vi "niFpga wdp fft butterfly.vi"(6 "enable":bool, 8 "index=0?":bool, 9 "twiddle factor":T1, 10 "data in 1":T2, 11 "data in 0":T2) -> (2 "data out 1":cluster{"y":fxp<+/-,11,2>, "y":fxp<+/-,11,2>}, 3 "data out 0":cluster{"y":fxp<+/-,11,2>, "y":fxp<+/-,11,2>})   [LabVIEW 2017]
uses:
  <vilib>/rvi/Analysis/measure/FFT/config/niFpgaFFTScalingScheme.ctl
  <vilib>/rvi/ClientSDK/Core/DevComputerLib/Private/FourWireProtocol(cint64).vi
  <vilib>/rvi/FXPMathLib/FxpAdd/XNode/nifxpmath_Add.xnode
  <vilib>/rvi/FXPMathLib/FxpSub/XNode/nifxpmath_Sub.xnode
  <vilib>/rvi/FXPMathLib/FxpMultComplex/XNode/niFpgaMultComplex.xnode
  <vilib>/rvi/FXPMathLib/SharedSubVIs/typedef/nifxpmath_BASIC_ImplementationSettings.ctl
  <vilib>/fxp/LVFixedPointQuantizationPolicyTypeDef.ctl
  <vilib>/fxp/LVFixedPointOverflowPolicyTypeDef.ctl
  <vilib>/rvi/FXPMathLib/FxpInterpret/XNode/nifxpmath_Interpret.xnode
  <vilib>/rvi/FXPMathLib/sim/FxpSim.dll
  <vilib>/rvi/ClientSDK/Core/DevComputerLib/niFpgaDevCompUtilities.lvlib
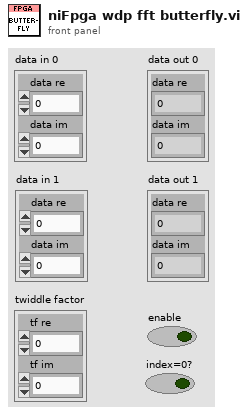
[diagram p1: front panel]
types:
  T1 = cluster{"tf re":fxp<+/-,16,2>, "tf im":fxp<+/-,16,2>}
  T2 = cluster{"data re":fxp<+/-,8,1>, "data im":fxp<+/-,8,1>}
  T3 = typedef "niFpgaFFTScalingScheme.ctl" = enum16{"Unscaled", "Scaled"}
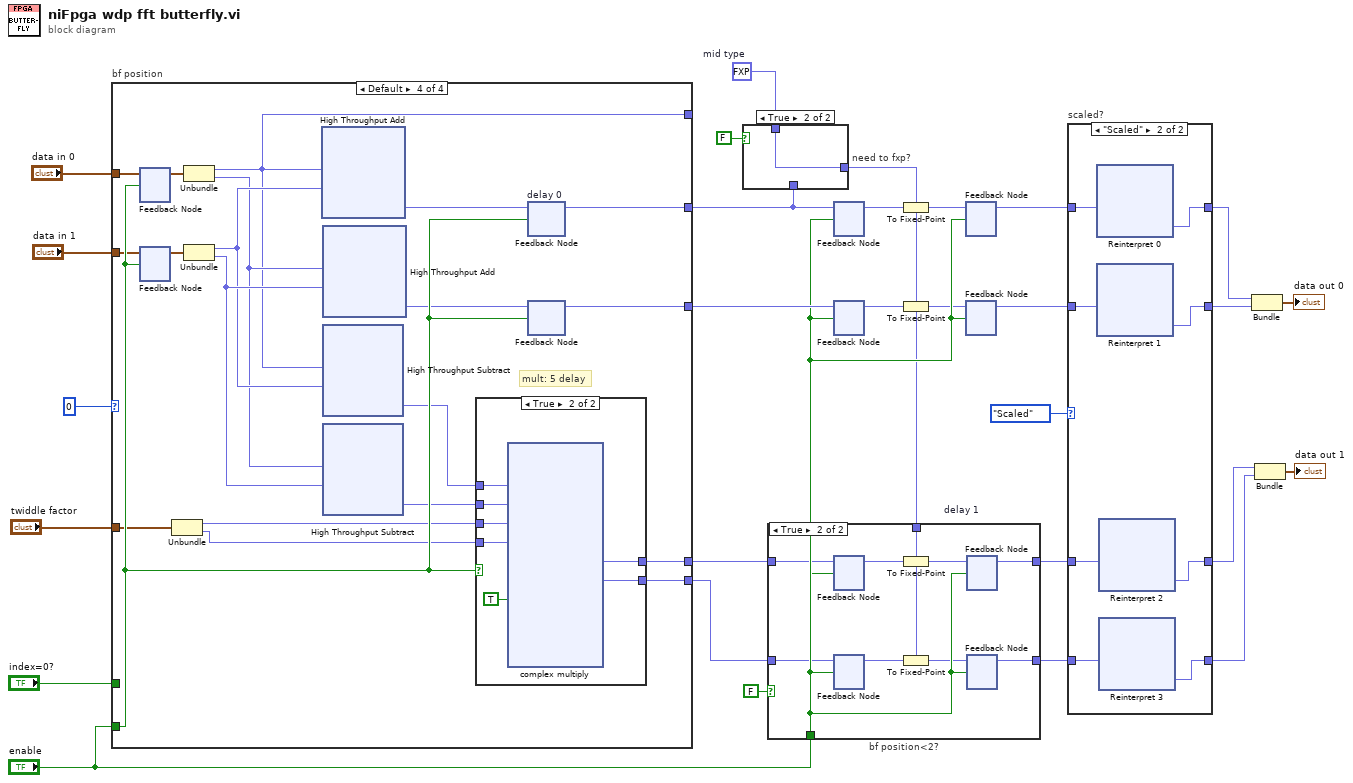
[diagram p0: block diagram]
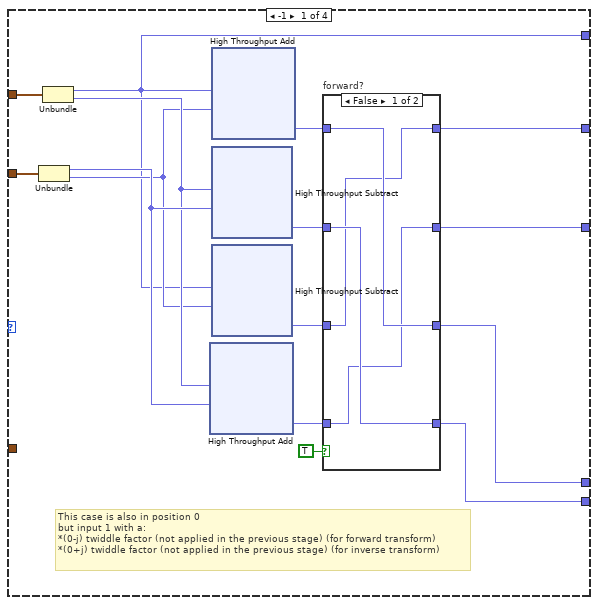
[diagram p5: hidden frame]
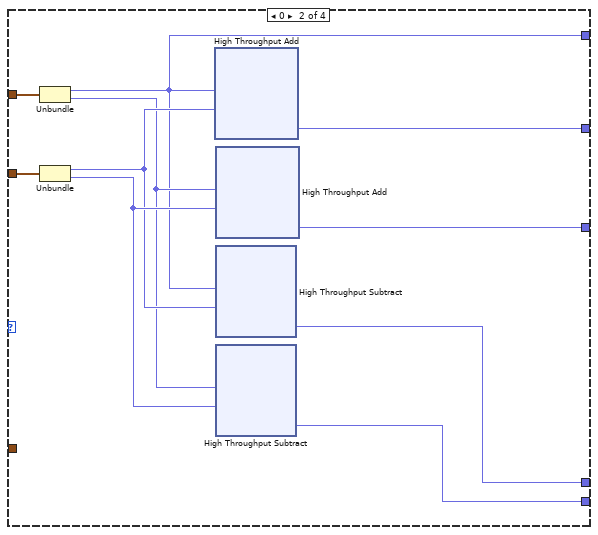
[diagram p7: hidden frame]
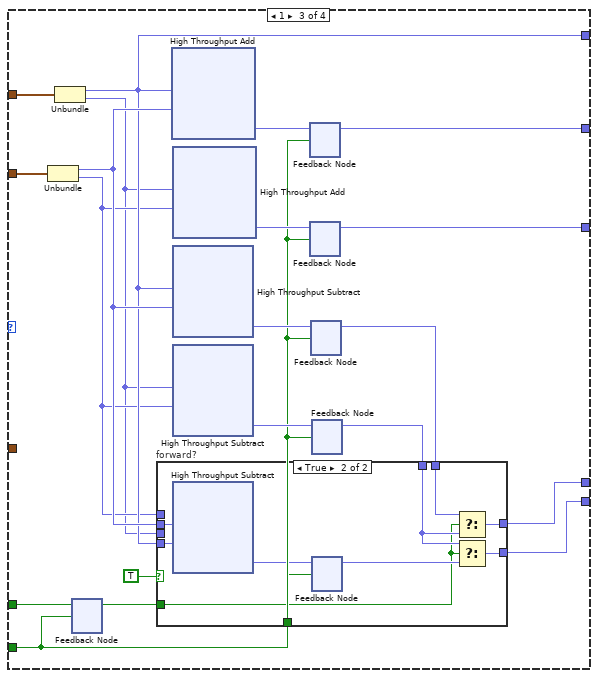
[diagram p8: hidden frame]
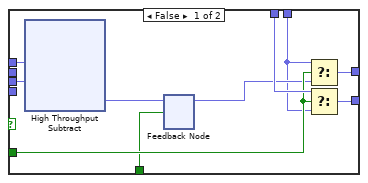
[diagram p9: hidden frame]
diagram:
  w24 = fxp<+/-,10,2> 0.0  # mid type
  n1 = case "bf position" shown="Default" 0 {
    tunnel: "enable" -> [_ _ w71 w122]
    tunnel: [w32 w53 w66 w121] -> w17
    tunnel: [w34 w54 w67 w120] -> w18
    tunnel: "twiddle factor" -> [_ _ _ w119]
    tunnel: "data in 1" -> [w40 w58 w73 w117]
    tunnel: "data in 0" -> [w41 w59 w74 w115]
    tunnel: [w38 w57 w69 w105] -> w29
    tunnel: [w36 w55 w68 w104] -> w28
    tunnel: [w39 w56 w70 w103] -> _
    tunnel: "index=0?" -> [_ _ w72 _]
    frame -1 {
      # "This case is also in position 0\nbut input 1 with a:\n*(0-j) twiddle factor (not applied in the previous stage) (for forward transform)\n*(0+j) twiddle factor (not applied in the previous stage) (for inverse transform)"
      n2 = Unbundle(w40) -> ("data re"=w44:fxp<+/-,8,1>, "data im"=w42:fxp<+/-,8,1>)
      n3 = Unbundle(w41) -> ("data re"=w39:fxp<+/-,8,1>, "data im"=w43:fxp<+/-,8,1>)
      n4 = xnode "High Throughput Add"("x"=w43, "y"=w44) -> ("x+y"=w31:fxp<+/-,9,2>)
      n5 = xnode "High Throughput Add"("x"=w39, "y"=w42) -> ("x+y"=w37:fxp<+/-,9,2>)
      n6 = xnode "High Throughput Subtract"("x"=w43, "y"=w44) -> ("x-y"=w35:fxp<+/-,9,2>)
      n7 = xnode "High Throughput Subtract"("x"=w39, "y"=w42) -> ("x-y"=w33:fxp<+/-,9,2>)
      n8 = case "forward?" shown="False" TRUE {
        tunnel: [w46 w52] -> w38
        tunnel: w37 -> [w48 w52]
        tunnel: [w45 w51] -> w36
        tunnel: w35 -> [w47 w51]
        tunnel: [w48 w50] -> w34
        tunnel: w33 -> [w46 w50]
        tunnel: [w47 w49] -> w32
        tunnel: w31 -> [w45 w49]
        frame False {
        }
        frame True {
        }
      }
    }
    frame 0 {
      n9 = Unbundle(w59) -> ("data re"=w56:fxp<+/-,8,1>, "data im"=w60:fxp<+/-,8,1>)
      n10 = Unbundle(w58) -> ("data re"=w61:fxp<+/-,8,1>, "data im"=w62:fxp<+/-,8,1>)
      n11 = xnode ("High Throughput Add")("x"=w56, "y"=w61) -> ("x+y"=w57:fxp<+/-,9,2>)
      n12 = xnode ("High Throughput Add")("x"=w60, "y"=w62) -> ("x+y"=w55:fxp<+/-,9,2>)
      n13 = xnode ("High Throughput Subtract")("x"=w56, "y"=w61) -> ("x-y"=w54:fxp<+/-,9,2>)
      n14 = xnode ("High Throughput Subtract")("x"=w60, "y"=w62) -> ("x-y"=w53:fxp<+/-,9,2>)
    }
    frame 1 {
      n15 = Unbundle(w73) -> ("data re"=w75:fxp<+/-,8,1>, "data im"=w64:fxp<+/-,8,1>)
      n16 = Unbundle(w74) -> ("data re"=w70:fxp<+/-,8,1>, "data im"=w63:fxp<+/-,8,1>)
      n17 = feedback #1() -> (w76:bool)  [unwired: 1 in]
      n18 = feedback-in #1(w72, w71) -> ()
      n19 = xnode ("High Throughput Add")("x"=w70, "y"=w75) -> ("x+y"=w77:fxp<+/-,9,2>)
      n20 = xnode ("High Throughput Add")("x"=w63, "y"=w64) -> ("x+y"=w78:fxp<+/-,9,2>)
      n21 = xnode ("High Throughput Subtract")("x"=w70, "y"=w75) -> ("x-y"=w79:fxp<+/-,9,2>)
      n22 = xnode ("High Throughput Subtract")("x"=w63, "y"=w64) -> ("x-y"=w81:fxp<+/-,9,2>)
      n23 = feedback #2() -> (w69:fxp<+/-,9,2>)  [unwired: 1 in]
      n24 = feedback-in #2(w77, w71) -> ()
      n25 = feedback #3() -> (w68:fxp<+/-,9,2>)  [unwired: 1 in]
      n26 = feedback-in #3(w78, w71) -> ()
      n27 = feedback #4() -> (w80:fxp<+/-,9,2>)  [unwired: 1 in]
      n28 = feedback-in #4(w79, w71) -> ()
      n29 = feedback #5() -> (w82:fxp<+/-,9,2>)  [unwired: 1 in]
      n30 = case "forward?" shown="True" TRUE {
        tunnel: w82 -> [w91 w100]
        tunnel: w80 -> [w83 w99]
        tunnel: w76 -> [w90 w98]
        tunnel: w75 -> [_ w97]
        tunnel: w71 -> [w89 w96]
        tunnel: w70 -> [_ w95]
        tunnel: [w88 w94] -> w67
        tunnel: [w87 w93] -> w66
        tunnel: w64 -> [w86 _]
        tunnel: w63 -> [w85 _]
        frame False {
          n31 = xnode ("High Throughput Subtract")("x"=w86, "y"=w85) -> ("x-y"=w92:fxp<+/-,9,2>)
          n32 = feedback #6() -> (w84:fxp<+/-,9,2>)  [unwired: 1 in]
          n33 = feedback-in #6(w92, w89) -> ()
          n34 = Select(t=w83, s=w90, f=w84) -> (s? t:f=w88:fxp<+/-,9,2>)
          n35 = Select(t=w91, s=w90, f=w83) -> (s? t:f=w87:fxp<+/-,9,2>)
        }
        frame True {
          n36 = xnode ("High Throughput Subtract")("x"=w97, "y"=w95) -> ("x-y"=w101:fxp<+/-,9,2>)
          n37 = feedback #7() -> (w102:fxp<+/-,9,2>)  [unwired: 1 in]
          n38 = feedback-in #7(w101, w96) -> ()
          n39 = Select(t=w99, s=w98, f=w100) -> (s? t:f=w94:fxp<+/-,9,2>)
          n40 = Select(t=w100, s=w98, f=w102) -> (s? t:f=w93:fxp<+/-,9,2>)
        }
      }
      n41 = feedback-in #5(w81, w71) -> ()
    }
    frame Default {
      # "mult: 5 delay"
      n42 = feedback #8() -> (w116:T2)  [unwired: 1 in]
      n43 = feedback-in #8(w115, w122) -> ()
      n44 = feedback #9() -> (w118:T2)  [unwired: 1 in]
      n45 = feedback-in #9(w117, w122) -> ()
      n46 = Unbundle(w119) -> ("tf re"=w109:fxp<+/-,16,2>, "tf im"=w110:fxp<+/-,16,2>)
      n47 = Unbundle(w116) -> ("data re"=w103:fxp<+/-,8,1>, "data im"=w106:fxp<+/-,8,1>)
      n48 = Unbundle(w118) -> ("data re"=w113:fxp<+/-,8,1>, "data im"=w114:fxp<+/-,8,1>)
      n49 = xnode ("High Throughput Add")("x"=w103, "y"=w113) -> ("x+y"=w107:fxp<+/-,9,2>)
      n50 = xnode ("High Throughput Add")("x"=w106, "y"=w114) -> ("x+y"=w108:fxp<+/-,9,2>)
      n51 = xnode ("High Throughput Subtract")("x"=w103, "y"=w113) -> ("x-y"=w111:fxp<+/-,9,2>)
      n52 = xnode ("High Throughput Subtract")("x"=w106, "y"=w114) -> ("x-y"=w112:fxp<+/-,9,2>)
      n53 = case shown="True" w122 {
        tunnel: w109 -> [_ w129]
        tunnel: w110 -> [_ w128]
        tunnel: [_ w127] -> w120
        tunnel: [_ w126] -> w121
        tunnel: w111 -> [_ w125]
        tunnel: w112 -> [_ w124]
        frame False {
        }
        frame True {
          n54 = xnode "complex multiply"("xr"=w125, "xi"=w124, "yr"=w129, "yi"=w128, "input valid"=TRUE) -> ("pr"=w127:fxp<+/-,9,2>, "pi"=w126:fxp<+/-,9,2>)  [unwired: 1 in, 2 out]
        }
      }
      n55 = feedback #10 "delay 0"() -> (w105:fxp<+/-,9,2>)  [unwired: 1 in]
      n56 = feedback-in #10(w107, w122) -> ()
      n57 = feedback #11 "delay 1"() -> (w104:fxp<+/-,9,2>)  [unwired: 1 in]
      n58 = feedback-in #11(w108, w122) -> ()
    }
  }
  n59 = case "need to fxp?" shown="True" FALSE {
    tunnel: [w249 w250] -> w12
    tunnel: w24 -> [_ w250]
    tunnel: w29 -> [w249 _]
    frame False {
    }
    frame True {
    }
  }
  n60 = case "bf position<2?" shown="True" FALSE {
    tunnel: "enable" -> [_ w262]
    tunnel: w18 -> [w252 w261]
    tunnel: w17 -> [w251 w260]
    tunnel: [w252 w257] -> w3
    tunnel: [w251 w255] -> w1
    tunnel: w12 -> [_ w253]
    frame False {
    }
    frame True {
      n61 = feedback #12() -> (w258:fxp<+/-,9,2>)  [unwired: 1 in]
      n62 = feedback-in #12(w261, w262) -> ()
      n63 = feedback #13() -> (w259:fxp<+/-,9,2>)  [unwired: 1 in]
      n64 = feedback-in #13(w260, w262) -> ()
      n65 = To Fixed-Point(fixed-point type=w253, number=w258) -> (fixed-point=w256:fxp<+/-,10,2>)
      n66 = To Fixed-Point(fixed-point type=w253, number=w259) -> (fixed-point=w254:fxp<+/-,10,2>)
      n67 = feedback #14() -> (w257:fxp<+/-,10,2>)  [unwired: 1 in]
      n68 = feedback-in #14(w256, w262) -> ()
      n69 = feedback #15() -> (w255:fxp<+/-,10,2>)  [unwired: 1 in]
      n70 = feedback-in #15(w254, w262) -> ()
    }
  }
  n71 = feedback #16() -> (w15:fxp<+/-,9,2>)  [unwired: 1 in]
  n72 = feedback-in #16(w29, "enable") -> ()
  n73 = feedback #17() -> (w16:fxp<+/-,9,2>)  [unwired: 1 in]
  n74 = feedback-in #17(w28, "enable") -> ()
  n75 = To Fixed-Point(fixed-point type=w12, number=w15) -> (fixed-point=w13:fxp<+/-,10,2>)
  n76 = To Fixed-Point(fixed-point type=w12, number=w16) -> (fixed-point=w14:fxp<+/-,10,2>)
  n77 = feedback #18() -> (w7:fxp<+/-,10,2>)  [unwired: 1 in]
  n78 = feedback-in #18(w13, "enable") -> ()
  n79 = feedback #19() -> (w5:fxp<+/-,10,2>)  [unwired: 1 in]
  n80 = feedback-in #19(w14, "enable") -> ()
  n81 = case "scaled?" shown="\"Scaled\"" niFpgaFFTScalingScheme."Scaled" {
    tunnel: [w266 w273] -> w8
    tunnel: w7 -> [w266 w274]
    tunnel: [w265 w271] -> w6
    tunnel: w5 -> [w265 w272]
    tunnel: [w264 w269] -> w4
    tunnel: w3 -> [w264 w270]
    tunnel: [w263 w267] -> w2
    tunnel: w1 -> [w263 w268]
    frame "Unscaled" {
    }
    frame "Scaled" {
      n82 = xnode "Reinterpret 0"("x"=w274) -> ("y"=w273:fxp<+/-,10,1>)
      n83 = xnode "Reinterpret 1"("x"=w272) -> ("y"=w271:fxp<+/-,10,1>)
      n84 = xnode "Reinterpret 2"("x"=w270) -> ("y"=w269:fxp<+/-,10,1>)
      n85 = xnode "Reinterpret 3"("x"=w268) -> ("y"=w267:fxp<+/-,10,1>)
    }
  }
  n86 = Bundle("y"=w8, "y"=w6) -> (→"data out 0":cluster{"y":fxp<+/-,11,2>, "y":fxp<+/-,11,2>})  [unwired: 1 in]
  n87 = Bundle("y"=w4, "y"=w2) -> (→"data out 1":cluster{"y":fxp<+/-,11,2>, "y":fxp<+/-,11,2>})  [unwired: 1 in]
